vi "AFM_Driver_Manager.OnLithographyFinish.vi"(8 "error in (no error)":errorcluster, 11 "AFM_Driver_Manager in":refnum<class "AFM_Driver_Manager.lvclass">) -> (0 "error out":errorcluster, 3 "AFM_Driver_Manager out":refnum<class "AFM_Driver_Manager.lvclass">)   [LabVIEW 2019, in "AFM_Driver_Manager.lvclass"]
uses:
  AFM_Driver_Manager.lvclass
  AFM_Driver_Manager.lvclass/AFM_Driver_Manager.ctl
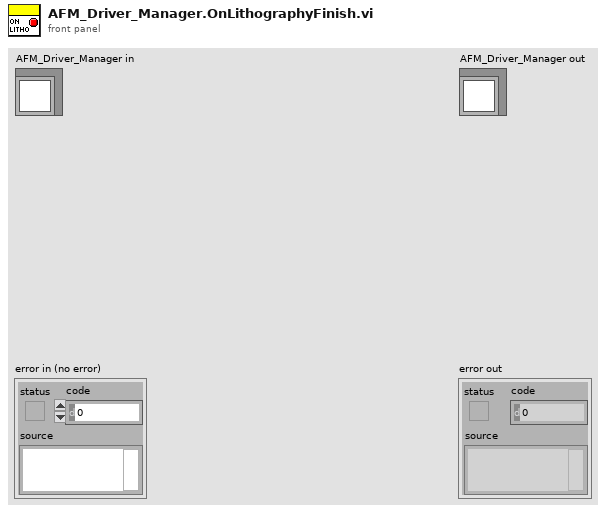
[diagram p1: front panel]
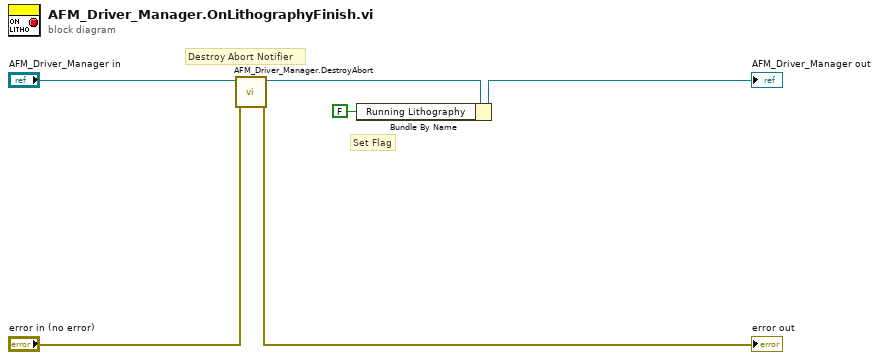
[diagram p0: block diagram]
diagram:
  # "Set Flag"
  # "Destroy Abort Notifier"
  n1 = call "AFM_Driver_Manager.DestroyAbort.vi"("error in (no error)"="error in (no error)", "AFM_Driver_Manager in"="AFM_Driver_Manager in") -> ("error out"=→"error out":errorcluster, "AFM_Driver_Manager out"=w2:refnum<class "AFM_Driver_Manager.lvclass">)  [unwired: 8 in]
  n2 = Bundle By Name(cluster=w2, "Running Lithography"=FALSE) -> (→"AFM_Driver_Manager out":refnum<class "AFM_Driver_Manager.lvclass">)
